vi "disconnect.vi"(8 "error in (no error)":errorcluster, 11 "py in":T1) -> (0 "error out":errorcluster)   [LabVIEW 2022 SP3, in "pythonq.lvlib"]
uses:
  pythonq.lvlib
  py_session.ctl
  py_cluster.ctl
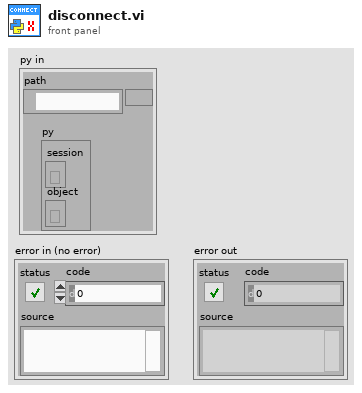
[diagram p1: front panel]
types:
  T1 = typedef "pythonq.lvlib/py_cluster.ctl" = cluster{"path":path, "py":T2}
  T2 = typedef "pythonq.lvlib/py_session.ctl" = cluster{"session":refnum<k35>, "object":refnum<k38>}
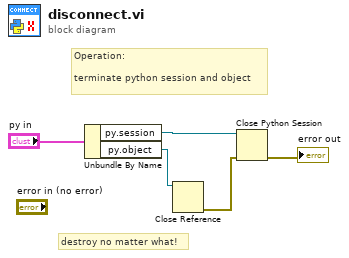
[diagram p0: block diagram]
diagram:
  # "Operation:\n\nterminate python session and object"
  # "destroy no matter what!"
  n1 = Unbundle By Name("py in") -> ("py.session"=w5:refnum<k35>, "py.object"=w3:refnum<k38>)
  n2 = Close Reference(reference=w3) -> (error out=w4:errorcluster)  [unwired: 1 in]
  n3 = Close Python Session(session in=w5, error in=w4) -> (11:→"error out":errorcluster)
